vi "get_test_output.vi"(7 "DAQmx Device Name":tag="Dev1", 8 "error in":errorcluster, 10 "Meas environment":T3) -> (0 "error out":errorcluster, 2 "Outputs":T2)   [LabVIEW 2024]
doc: "This VI performs a set of voltage measurements defined in the state machine as follows:\n- get Input V: performs a Measure Vin type measurement and saves the DC/RMS result as Input V avg\n- get Output V: performs a Measure Vout type measurement and saves the DC/RMS result as Output V avg, the Amplitude result as Output V ampl and based on the Rload_value Ohm environmental value calculates the Output Current\n- get Input Current: performs a Measure VRsense type measurement, and based on the ratio of DC/RMS result and the Rsense_value_Ohm environmental value saves the Input current\n- calc Efficency: calculates the input and output powers based on the output and input voltage and current values. As a ratio of output and input power the efficiency value is calculated and saved.\n- disable loads: deactivates the loads (all loads set to FALSE)\n-end"
uses:
  ctl_meas_env_cluster.ctl
  ctl_test_outputs_cluster.ctl
  ctl_get_test_output_states_enum.ctl
  ctl_volt_meas_modes_enum.ctl
  ctl_load_set_cluster.ctl
  <vilib>/measure/madcrms.llb/Basic Averaged DC-RMS for N Chan.vi
  <vilib>/measure/mascope.llb/Amplitude and Levels N chan.vi
  <vilib>/measure/NI_MAPro.lvlib
panel:
  out "Current state":T1
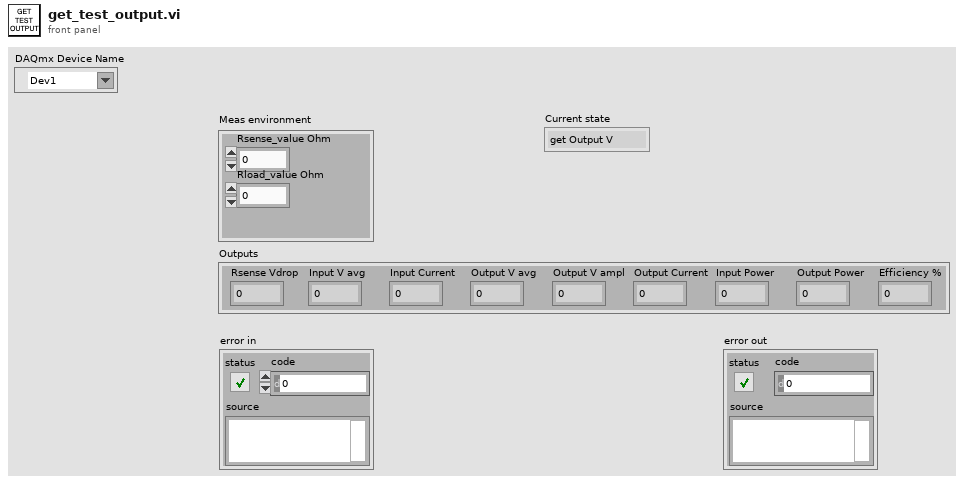
[diagram p1: front panel]
types:
  T1 = typedef "ctl_get_test_output_states_enum.ctl" = enum16{"get Output V", "get Input V", "get Input Current", "calc Efficiency", "disable loads", "end"}
  T2 = typedef "ctl_test_outputs_cluster.ctl" = cluster{"Output V avg":dbl, "Output V ampl":dbl, "Input Current":dbl, "Output Current":dbl, "Efficiency %":dbl, "Input V avg":dbl, "Input Power":dbl, "Output Power":dbl, "Rsense Vdrop":dbl}
  T3 = typedef "ctl_meas_env_cluster.ctl" = cluster{"Rsense_value Ohm":dbl, "Rload_value Ohm":dbl}
  T4 = typedef "ctl_voltage_meas_settings_cluster.ctl" = cluster{"Physical Channel":tag, "Min Voltage":dbl, "Max Voltage":dbl, "Terminal Configuration":i32, "Sample Rate":dbl, "Number of Samples":i32}
  T5 = typedef "ctl_volt_meas_modes_enum.ctl" = enum16{"Measure Vin", "Measure VRsense", "Measure Vout"}
  T6 = typedef "ctl_load_set_cluster.ctl" = cluster{"Resistor 1":bool, "Resistor 2":bool, "Resistor 3":bool, "Resistor 4":bool}
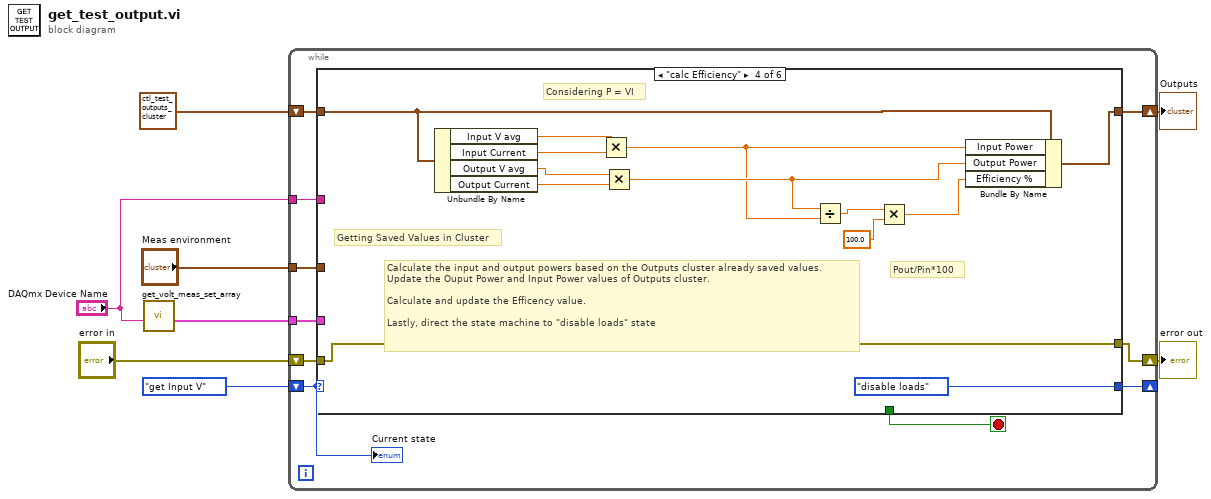
[diagram p0: block diagram]
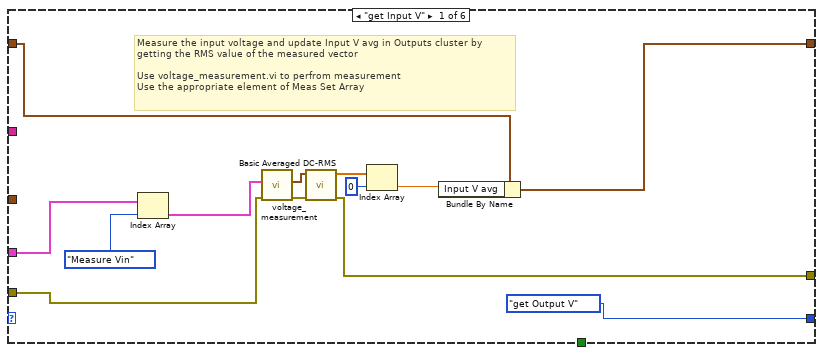
[diagram p2: hidden frame]
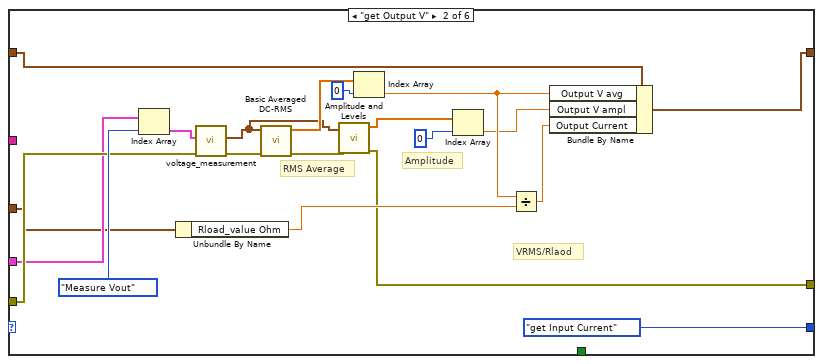
[diagram p3: hidden frame]
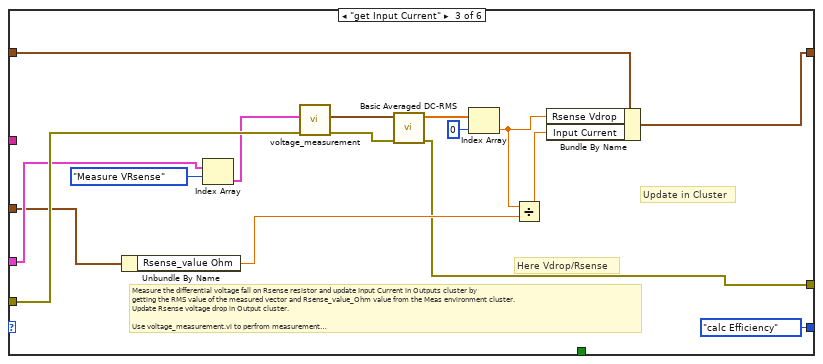
[diagram p4: hidden frame]
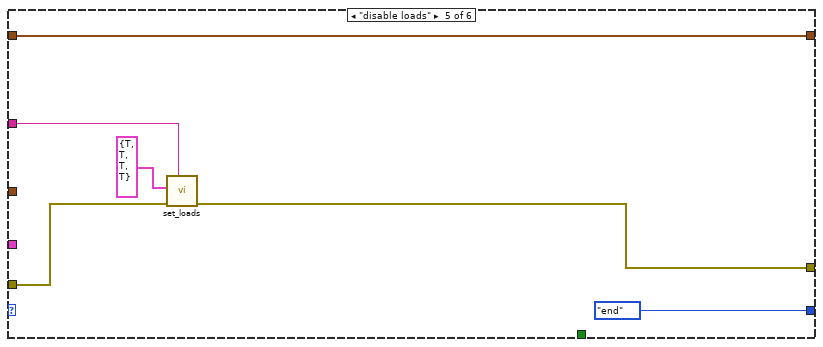
[diagram p5: hidden frame]
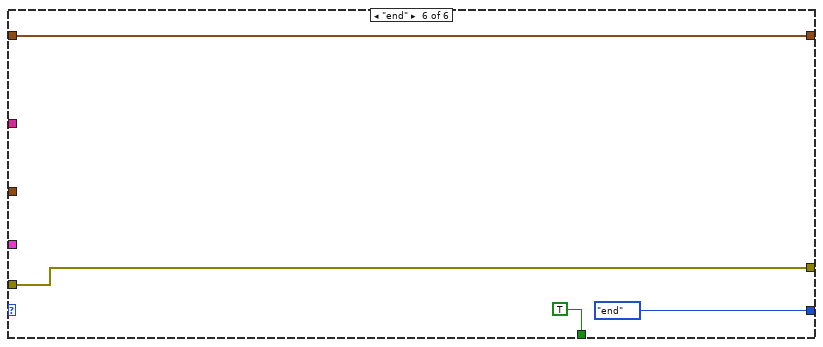
[diagram p6: hidden frame]
diagram:
  n1 = call "get_volt_meas_set_array.vi"("DAQmx Device Name"="DAQmx Device Name") -> ("Voltage meas settings array"=w5:T4[])  [unwired: 10 in]
  n2 = while {
    tunnel: "Meas environment" -> [w17]
    shift-right: [w11] -> _
    shift-left: ctl_get_test_output_states_enum."get Input V" -> [w18]
    shift-right: [w15] -> w3
    shift-left: T2 {"Output V avg"=0.0, "Output V ampl"=0.0, "Input Current"=0.0, "Output Current"=0.0, "Efficiency %"=0.0, "Input V avg"=0.0, "Input Power"=0.0, "Output Power"=0.0, "Rsense Vdrop"=0.0} ("Outputs") -> [w16]
    tunnel: w5 -> [w14]
    shift-right: [w13] -> w2
    shift-left: "error in" -> [w12]
    tunnel: "DAQmx Device Name" -> [w9]
    stop <- w10 stop-if-true
    n3 = case shown="\"calc Efficiency\"" w18 {
      tunnel: w17 -> [_ w41 w62 _ _ _]
      tunnel: w16 -> [w22 w46 w58 w79 w86 w90]
      tunnel: [w19 w37 w54 w68 w86 w90] -> w15
      tunnel: w14 -> [w30 w42 w65 _ _ _]
      tunnel: [w23 w35 w52 w78 w83 w88] -> w13
      tunnel: w12 -> [w29 w50 w67 w78 w84 w88]
      tunnel: [ctl_get_test_output_states_enum."get Output V" ctl_get_test_output_states_enum."get Input Current" ctl_get_test_output_states_enum."calc Efficiency" ctl_get_test_output_states_enum."disable loads" ctl_get_test_output_states_enum."end" ctl_get_test_output_states_enum."end"] -> w11
      tunnel: [_ _ _ _ _ TRUE] -> w10
      tunnel: w9 -> [_ _ _ _ w81 _]
      frame "get Input V" {
        # "Measure the input voltage and update Input V avg in Outputs cluster by\ngetting the RMS value of the measured vector\n\nUse voltage_measurement.vi to perfrom measurement\nUse the appropriate element of Meas Set Array"
        n4 = Index Array(array=w30, index=ctl_volt_meas_modes_enum."Measure Vin" ("Voltage meas modes")) -> (element=w27:T4)
        n5 = call "voltage_measurement.vi"("error in"=w29, "Voltage meas settings"=w27) -> ("error out"=w26:errorcluster, "Waveform Graph"=w25:waveform(dbl)[])  [unwired: 8 in]
        n6 = call-poly <vilib>:"Basic Averaged DC-RMS.vi"("error in (no error)"=w26, "signals in"=w25) -> ("error out"=w23:errorcluster, "DC values"=w24:dbl[])  [unwired: 6 in, 2 out]
        n7 = Index Array(array=w24, index=0) -> (element=w21:dbl)
        n8 = Bundle By Name(cluster=w22, "Input V avg"=w21) -> (w19:T2)
      }
      frame "get Output V" {
        # "VRMS/Rlaod"
        # "Amplitude"
        # "RMS Average"
        n9 = Index Array(array=w42, index=ctl_volt_meas_modes_enum."Measure Vout" ("Voltage meas modes")) -> (element=w48:T4)
        n10 = Unbundle By Name(w41) -> ("Rload_value Ohm"=w40:dbl)
        n11 = call "voltage_measurement.vi"("error in"=w50, "Voltage meas settings"=w48) -> ("error out"=w49:errorcluster, "Waveform Graph"=w34:waveform(dbl)[])  [unwired: 8 in]
        n12 = call-poly <vilib>:"Basic Averaged DC-RMS.vi"("error in (no error)"=w49, "signals in"=w34) -> ("error out"=w36:errorcluster, "DC values"=w47:dbl[])  [unwired: 6 in, 2 out]
        n13 = call-poly <vilib>:"Amplitude and Levels.vi"("error in (no error)"=w36, "signal(s) in"=w34) -> ("error out"=w35:errorcluster, "amplitude"=w33:dbl[])  [unwired: 6 in, 2 out]
        n14 = Index Array(array=w47, index=0) -> (element=w38:dbl)
        n15 = Index Array(array=w33, index=0) -> (element=w32:dbl)
        n16 = Divide(x=w38, y=w40) -> (x/y=w39:dbl)
        n17 = Bundle By Name(cluster=w46, "Output V avg"=w38, "Output V ampl"=w32, "Output Current"=w39) -> (w37:T2)
      }
      frame "get Input Current" {
        # "Measure the differential voltage fall on Rsense resistor and update Input Current in Outputs cluster by\ngetting the RMS value of the measured vector and Rsense_value_Ohm value from the Meas environment cluster.\nUpdate Rsense voltage drop in Output cluster.\n\nUse voltage_measurement.vi to perfrom measurement\nUse the appropriate element of Meas Set Array"
        # "Update in Cluster"
        # "Here Vdrop/Rsense"
        n18 = Unbundle By Name(w62) -> ("Rsense_value Ohm"=w56:dbl)
        n19 = Index Array(array=w65, index=ctl_volt_meas_modes_enum."Measure VRsense" ("Voltage meas modes")) -> (element=w64:T4)
        n20 = call "voltage_measurement.vi"("error in"=w67, "Voltage meas settings"=w64) -> ("error out"=w53:errorcluster, "Waveform Graph"=w61:waveform(dbl)[])  [unwired: 8 in]
        n21 = call-poly <vilib>:"Basic Averaged DC-RMS.vi"("error in (no error)"=w53, "signals in"=w61) -> ("error out"=w52:errorcluster, "DC values"=w60:dbl[])  [unwired: 6 in, 2 out]
        n22 = Index Array(array=w60, index=0) -> (element=w57:dbl)
        n23 = Divide(x=w57, y=w56) -> (x/y=w55:dbl)
        n24 = Bundle By Name(cluster=w58, "Rsense Vdrop"=w57, "Input Current"=w55) -> (w54:T2)
      }
      frame "calc Efficiency" {
        # "Calculate the input and output powers based on the Outputs cluster already saved values.\nUpdate the Ouput Power and Input Power values of Outputs cluster.\n\nCalculate and update the Efficency value.\n\nLastly, direct the state machine to \"disable loads\" state"
        # "Pout/Pin*100"
        # "Considering P = VI"
        # "Getting Saved Values in Cluster"
        n25 = Unbundle By Name(w79) -> ("Input V avg"=w77:dbl, "Input Current"=w76:dbl, "Output V avg"=w75:dbl, "Output Current"=w74:dbl)
        n26 = Multiply(x=w77, y=w76) -> (x*y=w72:dbl)
        n27 = Multiply(x=w75, y=w74) -> (x*y=w73:dbl)
        n28 = Divide(x=w73, y=w72) -> (x/y=w71:dbl)
        n29 = Multiply(x=w71, y=100.0) -> (x*y=w69:dbl)
        n30 = Bundle By Name(cluster=w79, "Input Power"=w72, "Output Power"=w73, "Efficiency %"=w69) -> (w68:T2)
      }
      frame "disable loads" {
        n31 = call "set_loads.vi"("DAQmx Device Name"=w81, "error in"=w84, "Load Set"=T6 {"Resistor 1"=TRUE, "Resistor 2"=TRUE, "Resistor 3"=TRUE, "Resistor 4"=TRUE}) -> ("error out"=w83:errorcluster)  [unwired: 8 in]
      }
      frame "end" {
      }
    }
    "Current state" <- w18
  }
  "Outputs" <- w3
  "error out" <- w2
